vi "EnableDisable.vi"(8 "error in (no error)":errorcluster, 10 "Action":T1, 11 "MotorController in":refnum<class "MotorController.lvclass">) -> (0 "error out":errorcluster, 3 "MotorController out":refnum<class "MotorController.lvclass">)   [LabVIEW 2019, in "MotorController.lvclass"]
uses:
  MotorController.lvclass
  enable_disable_enum_typedef.ctl
  MotorController.lvclass/MotorController.ctl
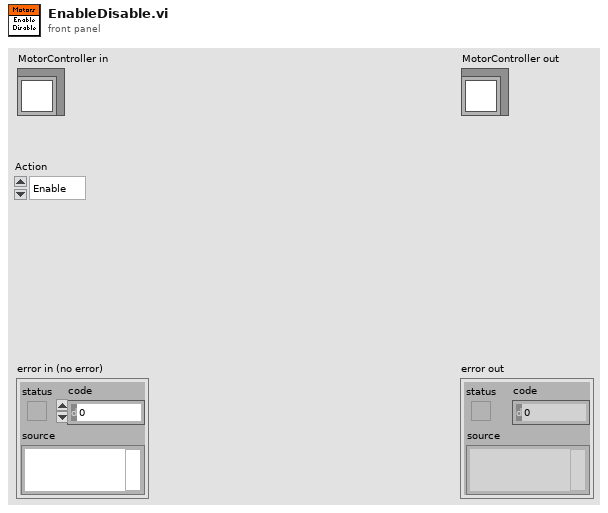
[diagram p1: front panel]
types:
  T1 = typedef "MotorController.lvclass/enable_disable_enum_typedef.ctl" = enum16{"Enable", "Disable"}
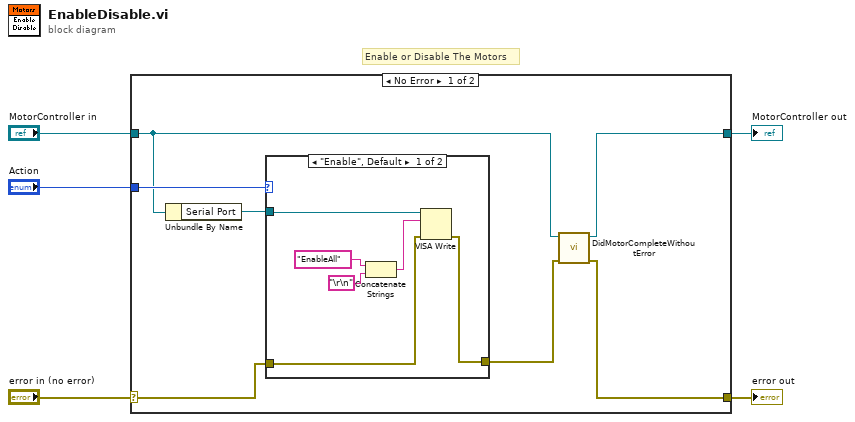
[diagram p0: block diagram]
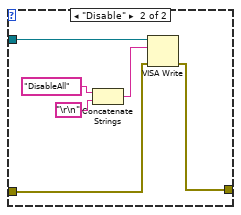
[diagram p2: hidden frame]
diagram:
  # "Enable or Disable The Motors"
  n1 = case shown="No Error" "error in (no error)" {
    selector: "error in (no error)" -> [w10 w26]
    tunnel: [w6 w26] -> w4
    tunnel: [w8 w25] -> w2
    tunnel: "MotorController in" -> [w9 w25]
    tunnel: "Action" -> [w12 _]
    frame No Error {
      n2 = Unbundle By Name(w9) -> ("Serial Port"=w11:refnum<visa-resource-name>)
      n3 = case shown="\"Enable\", Default" w12 {
        tunnel: w11 -> [w15 w24]
        tunnel: w10 -> [w13 w20]
        tunnel: [w14 w19] -> w7
        frame "Enable", Default {
          n4 = Concatenate Strings("EnableAll", "\r\n") -> (w18:string)
          n5 = VISA Write(VISA resource name=w15, write buffer=w18, error in (no error)=w13) -> (error out=w14:errorcluster)  [unwired: 2 out]
        }
        frame "Disable" {
          n6 = Concatenate Strings("DisableAll", "\r\n") -> (w21:string)
          n7 = VISA Write(VISA resource name=w24, write buffer=w21, error in (no error)=w20) -> (error out=w19:errorcluster)  [unwired: 2 out]
        }
      }
      n8 = call "DidMotorCompleteWithoutError.vi"("error in (no error)"=w7, "MotorController in"=w9) -> ("error out"=w6:errorcluster, "MotorController out"=w8:refnum<class "MotorController.lvclass">)  [unwired: 7 in, 1 out]
    }
    frame Error {
    }
  }
  "error out" <- w4
  "MotorController out" <- w2
